vi "fromXml.vi"(8 "error in (no error)":errorcluster, 10 "dataPointXml":refnum<class "xmlNode.lvclass">, 11 "DataPointScript in":refnum<class "DataPointScript.lvclass">) -> (0 "error out":errorcluster, 3 "DataPointScript out":refnum<class "DataPointScript.lvclass">)   [LabVIEW 2009, in "Tools.lvlib" / "Scripting.lvlib" / "DataPointScript.lvclass"]
uses:
  DataPointScript.lvclass
  xmlNode/xmlNode.lvclass
  ScriptingEvent/ScriptEvents/SingleToneArray/SingleToneArray.lvclass
  ScriptingEvent/ScriptEventList/ScriptEventList.lvclass
  DataPointScript.lvclass/DataPointScript.ctl
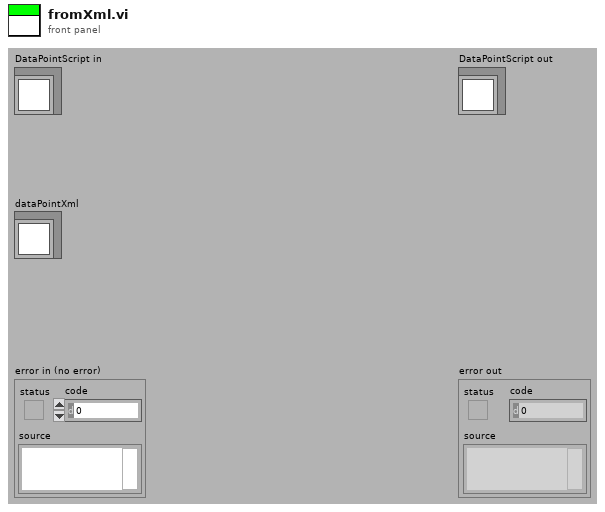
[diagram p1: front panel]
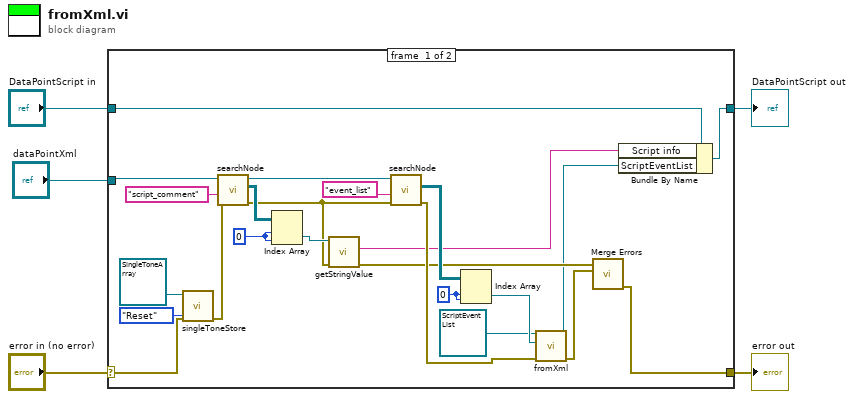
[diagram p0: block diagram]
diagram:
  n1 = case shown="No Error" "error in (no error)" {
    selector: "error in (no error)" -> [w7 w31]
    tunnel: [w14 w31] -> w4
    tunnel: [w10 w30] -> w2
    tunnel: "DataPointScript in" -> [w11 w30]
    tunnel: "dataPointXml" -> [w29 _]
    frame #0 {
      w21 = 0
      w24 = 0
      n2 = call "singleToneStore.vi"("error in (no error)"=w7, "action"=enum16{"Write", "Read", "Reset"}."Reset", "SingleToneArray in"=refnum<class "SingleToneArray.lvclass"> refnum) -> ("error out"=w6:errorcluster)  [unwired: 5 in, 3 out]
      n3 = call-dynamic "searchNode.vi"("error in (no error)"=w6, "searchElementName"="script_comment", "xmlNode in"=w29) -> ("error out"=w23:errorcluster, "arrayXmlNodes"=w26:refnum<class "xmlNode.lvclass">[][], "xmlNode out"=w27:refnum<class "xmlNode.lvclass">)  [unwired: 6 in]
      n4 = Index Array(array=w26, index (row)=w24, index (col)=w24) -> (element=w25:refnum<class "xmlNode.lvclass">)
      n5 = call-dynamic "getStringValue.vi"("error in (no error)"=w23, "xmlNode.lvclass in"=w25) -> ("error out"=w16:errorcluster, "stringValue"=w13:string)  [unwired: 7 in, 1 out]
      n6 = call-dynamic "searchNode.vi"("error in (no error)"=w23, "searchElementName"="event_list", "xmlNode in"=w27) -> ("error out"=w17:errorcluster, "arrayXmlNodes"=w20:refnum<class "xmlNode.lvclass">[][])  [unwired: 6 in, 1 out]
      n7 = Index Array(array=w20, index (row)=w21, index (col)=w21) -> (element=w19:refnum<class "xmlNode.lvclass">)
      n8 = call "fromXml.vi"("error in (no error)"=w17, "eventListXml"=w19, "ScriptEventList in"=refnum<class "ScriptEventList.lvclass"> refnum ("Tools.lvlib:Scripting.lvlib:ScriptEventList.lvclass")) -> ("error out"=w15:errorcluster, "ScriptEventList out"=w12:refnum<class "ScriptEventList.lvclass">)  [unwired: 7 in]
      n9 = call <vilib>:"Merge Errors.vi"("error in 2 (no error)"=w15, "error in 1 (no error)"=w16) -> ("error out"=w14:errorcluster)  [unwired: 5 in]
      n10 = Bundle By Name(cluster=w11, "Script info"=w13, "ScriptEventList"=w12) -> (w10:refnum<class "DataPointScript.lvclass">)
    }
    frame #1 {
    }
  }
  "error out" <- w4
  "DataPointScript out" <- w2
